vi "GUI - Template.vi"(5 "error in (no error)":errorcluster, 6 "ReInit All to Default?":bool, 7 "Application Name":string="GenUtil", 9 "State Queue":T1[](array[typedef])=["SC >>> Initialize"]) -> (19 "error out":errorcluster)   [LabVIEW 2020, in "Generic Utilities.lvclass"]
uses:
  Generic Utilities.lvclass
  utils/GenUtil State List.ctl
  <vilib>/Utility/sysdir.llb/System Directory Type.ctl
  <vilib>/Platform/browser.llb/Open URL in Default Browser (path).vi
  <vilib>/addons/_AddQ/G#Object/G#Object.lvclass
panel:
  in  "Task":enum32{"Monitor", "Settings"}(tab)
  in  "AppData Folder":bool
  out "State History":string[](array[string])
  out "State Index":i32
  out "Exec Time":dbl
  in  "TimeOut":i32=-1 caption="msec"
  in  "State 1":bool
  in  "Exit":bool
  # "Ó 2016"
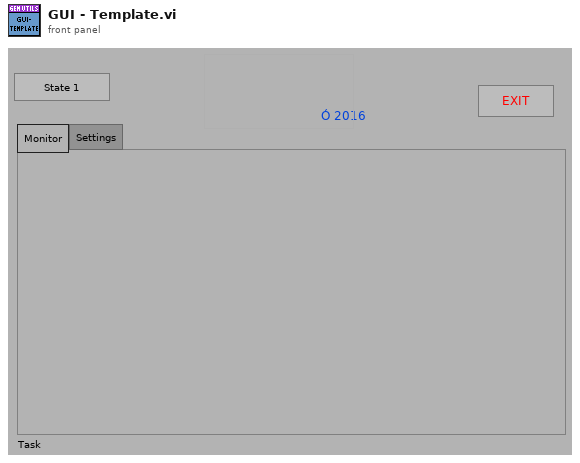
[diagram p1: front panel]
types:
  T1 = typedef "Generic Utilities.lvclass/GenUtil State List.ctl" = string
  T2 = enum32{"Invalid", "Standard", "Closed", "Hidden", "Minimized", "Maximized"}
  T3 = typedef "System Directory Type.ctl" = i32
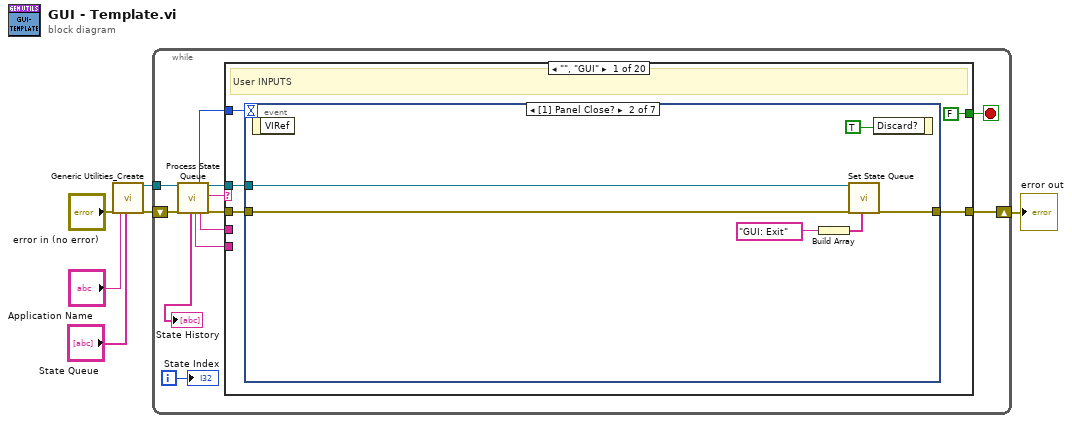
[diagram p0: block diagram]
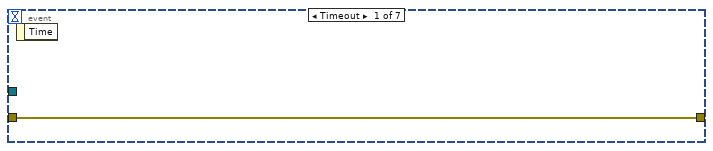
[diagram p2: hidden frame]
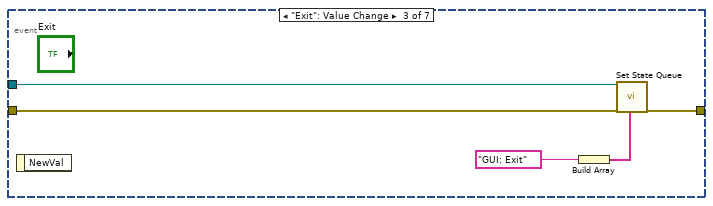
[diagram p3: hidden frame]
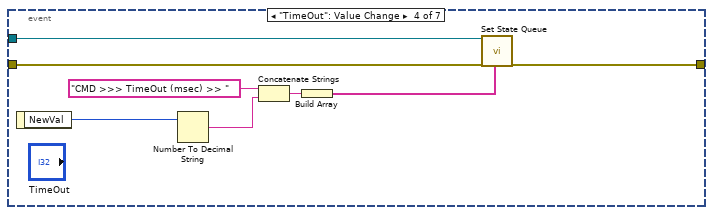
[diagram p4: hidden frame]
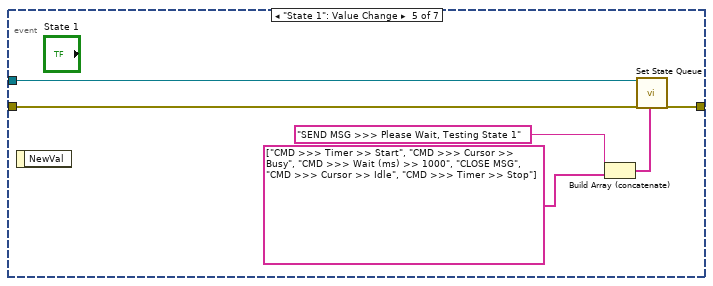
[diagram p5: hidden frame]
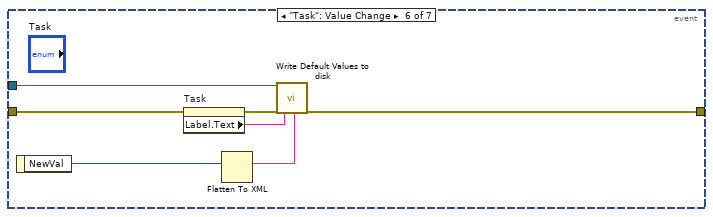
[diagram p6: hidden frame]
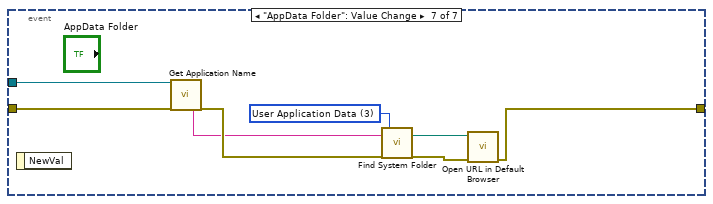
[diagram p7: hidden frame]
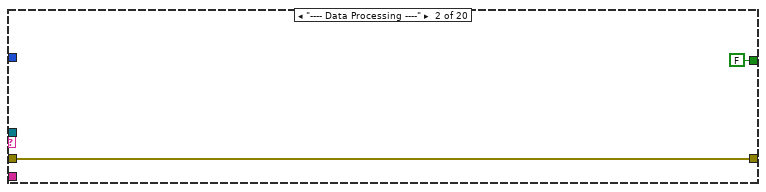
[diagram p8: hidden frame]
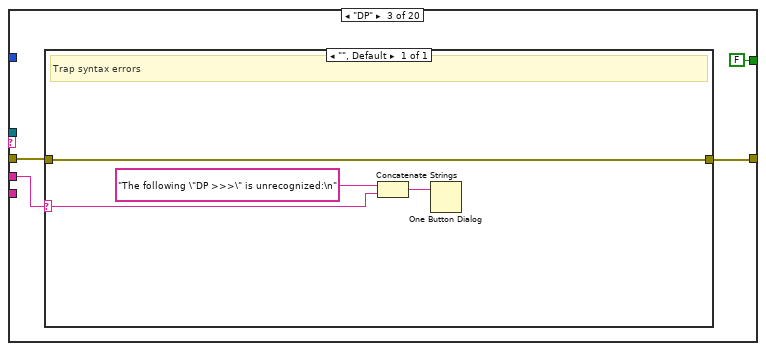
[diagram p9: hidden frame]
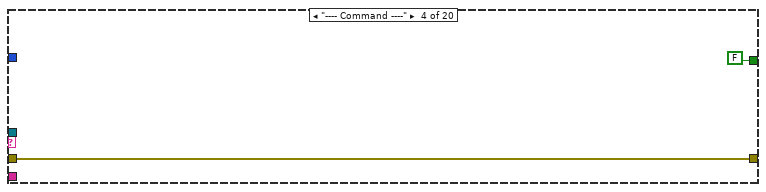
[diagram p10: hidden frame]
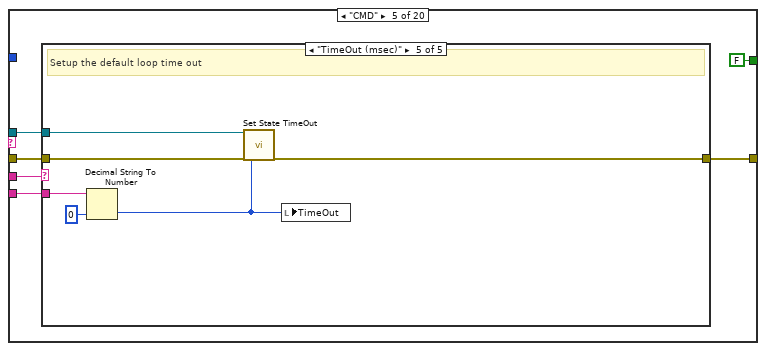
[diagram p11: hidden frame]
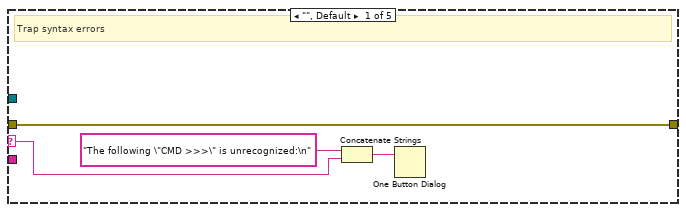
[diagram p12: hidden frame]
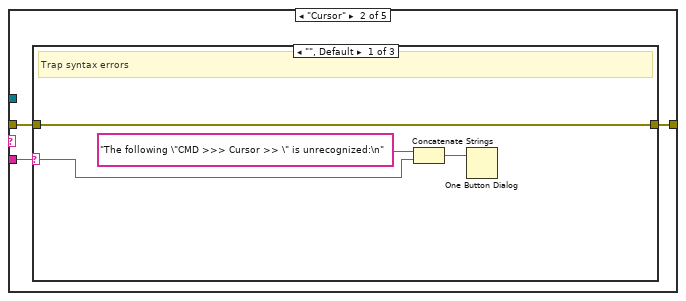
[diagram p13: hidden frame]
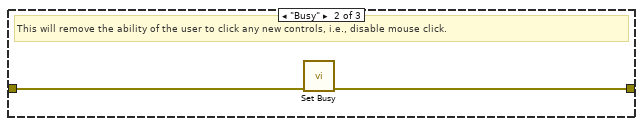
[diagram p14: hidden frame]
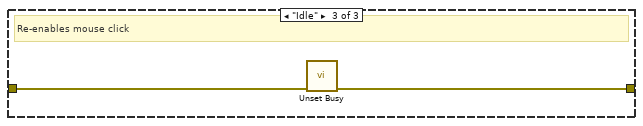
[diagram p15: hidden frame]
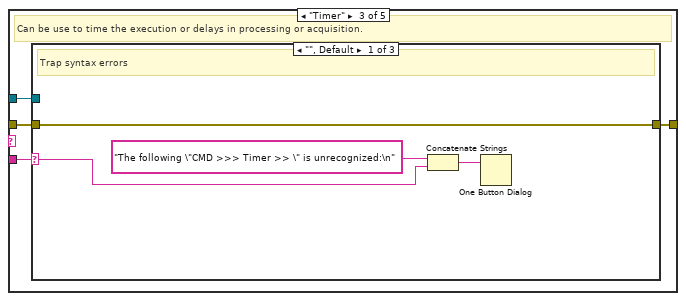
[diagram p16: hidden frame]
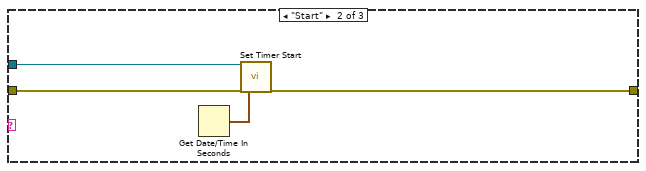
[diagram p17: hidden frame]
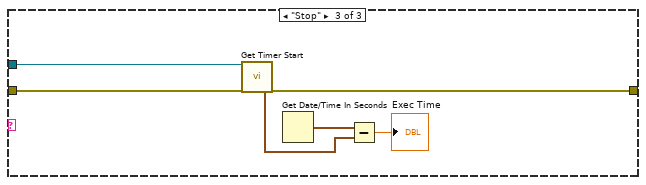
[diagram p18: hidden frame]
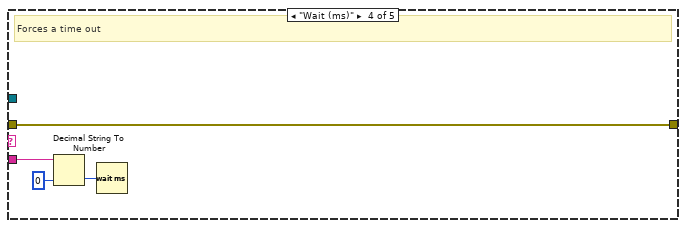
[diagram p19: hidden frame]
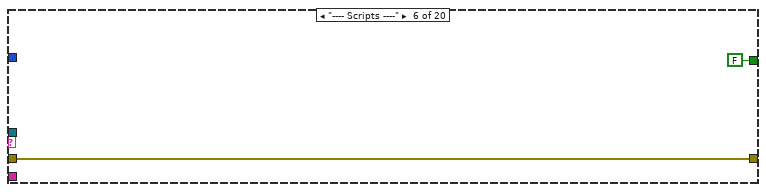
[diagram p20: hidden frame]
diagram:
  n1 = call "Generic Utilities_Create.vi"("error in (no error)"="error in (no error)", "Application Name"="Application Name", "State Queue"="State Queue") -> ("reference out"=w6:refnum<class "Generic Utilities.lvclass">, "error out"=w5:errorcluster)  [unwired: 15 in]
  n2 = while {
    shift-right: [w10] -> w1
    shift-left: w5 -> [w15]
    tunnel: w6 -> [w16]
    i -> [w17]
    stop <- w18 stop-if-true
    n3 = call "Process State Queue.vi"("reference in"=w16, "error in (no error)"=w15) -> ("State History"=→"State History":string[], "Additional Options"=w7:string, "Timeout"=w14:i32, "State Option"=w9:string, "reference out"=w13:refnum<class "Generic Utilities.lvclass">, "Current State"=w12:string, "error out"=w11:errorcluster)  [unwired: 10 in, 1 out]
    n4 = case shown="\"\", \"GUI\"" w12 {
      selector: w12 -> [_ _ _ _ _ _ _ _ _ _ _ _ _ _ _ _ w259 _ _ _]
      tunnel: w13 -> [w21 _ _ _ w77 _ w133 _ w144 w169 _ w199 w213 w248 w252 _ _ _ _ w269]
      tunnel: [FALSE FALSE FALSE FALSE FALSE FALSE FALSE FALSE FALSE FALSE FALSE FALSE TRUE FALSE FALSE FALSE FALSE FALSE FALSE TRUE] -> w18
      tunnel: w14 -> [w22 _ _ _ _ _ _ _ _ _ _ _ _ _ _ _ _ _ _ _]
      tunnel: w9 -> [_ _ w69 _ w81 _ w129 _ w145 w166 _ _ _ w245 _ _ _ _ _ _]
      tunnel: w11 -> [w20 w65 w68 w75 w79 w126 w132 w140 w142 w168 w189 w195 w210 w247 w253 w255 w257 w262 w265 w268]
      tunnel: [w19 w65 w67 w75 w80 w126 w131 w140 w143 w167 w189 w196 w209 w246 w251 w255 w257 errorcluster {"status"=FALSE, "code"=0, "source"=""} ("error out") w265 w267] -> w10
      tunnel: w7 -> [_ _ _ _ w78 _ _ _ _ _ _ _ _ _ _ _ _ _ _ _]
      frame "", "GUI" {
        # "User INPUTS"
        n5 = event shown="[1] Panel Close?" {
          selector: _ -> [_ _ _ _ _ _ _]
          dyn-events: _ -> [_ _ _ _ _ _ _]
          timeout: w22 -> [_ _ _ _ _ _ _]
          tunnel: w21 -> [_ w29 w35 w39 w48 w55 w63]
          tunnel: w20 -> [w24 w28 w33 w38 w47 w52 w62]
          tunnel: [w24 w27 w34 w37 w49 w50 w57] -> w19
          event Timeout {
            n6 = event-data() -> ()  [unwired: 1 in, 1 out]
          }
          event Panel Close? {
            n7 = event-data() -> ()  [unwired: 1 in, 1 out]
            n8 = Build Array(T1 "GUI: Exit" ("State List")) -> (w26:T1[])
            n9 = call "Set State Queue.vi"("reference in"=w29, "error in (no error)"=w28, "State Queue"=w26) -> ("error out"=w27:errorcluster)  [unwired: 15 in, 1 out]
            n10 = event-data("Discard?"=TRUE) -> ()  [unwired: 1 in, 1 out]
          }
          event "Exit": Value Change {
            n11 = event-data() -> ()  [unwired: 1 in, 1 out]
            n12 = Build Array(T1 "GUI: Exit" ("State List")) -> (w32:T1[])
            n13 = call "Set State Queue.vi"("reference in"=w35, "error in (no error)"=w33, "State Queue"=w32) -> ("error out"=w34:errorcluster)  [unwired: 15 in, 1 out]
          }
          event "TimeOut": Value Change {
            n14 = event-data() -> ("NewVal"=w36:i32)  [unwired: 1 in]
            n15 = Number To Decimal String(number=w36) -> (decimal integer string=w41:string)  [unwired: 1 in]
            n16 = Concatenate Strings("CMD >>> TimeOut (msec) >> " ("String"), w41) -> (w42:string)
            n17 = Build Array(w42) -> (w43:string[])
            n18 = call "Set State Queue.vi"("reference in"=w39, "error in (no error)"=w38, "State Queue"=w43) -> ("error out"=w37:errorcluster)  [unwired: 15 in, 1 out]
          }
          event "State 1": Value Change {
            n19 = event-data() -> ()  [unwired: 1 in, 1 out]
            n20 = Build Array (concatenate)("SEND MSG >>> Please Wait, Testing State 1" ("String"), T1[] ["CMD >>> Timer >> Start", "CMD >>> Cursor >> Busy", "CMD >>> Wait (ms) >> 1000", "CLOSE MSG", "CMD >>> Cursor >> Idle", "CMD >>> Timer >> Stop"] ("State Queue OUT")) -> (w44:T1[])
            n21 = call "Set State Queue.vi"("reference in"=w48, "error in (no error)"=w47, "State Queue"=w44) -> ("error out"=w49:errorcluster)  [unwired: 15 in, 1 out]
          }
          event "Task": Value Change {
            n22 = event-data() -> ("NewVal"=w56:enum32{"Monitor", "Settings"})  [unwired: 1 in]
            n23 = property on="Task" class="TabCtl (strict)"(error in=w52) -> (error out=w51:errorcluster, "Label.Text"=w54:string)  [unwired: 1 in, 1 out]
            n24 = Flatten To XML(6:w56) -> (2:w53:string)
            n25 = call-dynamic "Write Default Values to disk.vi"("reference in"=w55, "error in (no error)"=w51, "Control Label"=w54, "Value (XML String)"=w53) -> ("error out"=w50:errorcluster)  [unwired: 14 in, 1 out]
          }
          event "AppData Folder": Value Change {
            w64 = T3 3 items=["User Home"=0, "User Desktop"=1, "User Documents"=2, "User Application Data"=3, "User Preferences"=4, "User Temporary"=5, "Public Documents"=6, "Public Application Data"=7, "Public Preferences"=8, "Public Cache"=13, "System Core Libraries"=9, "System Installed Libraries"=10, "Application Files"=11, "Boot Volume Root"=12] ("system directory type")
            n26 = event-data() -> ()  [unwired: 1 in, 1 out]
            n27 = call "Get Application Name.vi"("reference in"=w63, "error in (no error)"=w62) -> ("Application Name"=w60:string, "error out"=w61:errorcluster)  [unwired: 15 in, 1 out]
            n28 = call "Find System Folder.vi"("Application Name"=w60, "error in (no error)"=w61, "system directory type"=w64) -> ("System Folder"=w59:path, "error out"=w58:errorcluster)  [unwired: 15 in]
            n29 = call-poly <vilib>:"Open URL in Default Browser.vi"("error in (no error)"=w58, "path"=w59) -> ("error out"=w57:errorcluster)  [unwired: 4 in, 1 out]
          }
        }
      }
      frame "---- Data Processing ----" {
      }
      frame "DP" {
        n30 = case shown="\"\", Default" w69 {
          selector: w69 -> [w72]
          tunnel: [w71] -> w67
          tunnel: w68 -> [w71]
          frame "", Default {
            # "Trap syntax errors"
            n31 = Concatenate Strings("The following \"DP >>>\" is unrecognized:\n", w72) -> (w73:string)
            n32 = One Button Dialog(message=w73) -> ()  [unwired: 1 in, 1 out]
          }
        }
      }
      frame "---- Command ----" {
      }
      frame "CMD" {
        n33 = case shown="\"TimeOut (msec)\"" w81 {
          selector: w81 -> [w84 _ _ _ _]
          tunnel: [w83 w88 w100 w119 w121] -> w80
          tunnel: w79 -> [w83 w87 w99 w119 w122]
          tunnel: w78 -> [_ w89 w101 w116 w124]
          tunnel: w77 -> [_ _ w98 _ w123]
          frame "", Default {
            # "Trap syntax errors"
            n34 = Concatenate Strings("The following \"CMD >>>\" is unrecognized:\n", w84) -> (w85:string)
            n35 = One Button Dialog(message=w85) -> ()  [unwired: 1 in, 1 out]
          }
          frame "Cursor" {
            n36 = case shown="\"\", Default" w89 {
              selector: w89 -> [w91 _ _]
              tunnel: [w90 w94 w96] -> w88
              tunnel: w87 -> [w90 w95 w97]
              frame "", Default {
                # "Trap syntax errors"
                n37 = Concatenate Strings("The following \"CMD >>> Cursor >> \" is unrecognized:\n", w91) -> (w92:string)
                n38 = One Button Dialog(message=w92) -> ()  [unwired: 1 in, 1 out]
              }
              frame "Busy" {
                # "This will remove the ability of the user to click any new controls, i.e., disable mouse click."
                n39 = call <vilib>:"Set Busy.vi"("error in (no error)"=w95) -> ("error out"=w94:errorcluster)  [unwired: 9 in, 1 out]
              }
              frame "Idle" {
                # "Re-enables mouse click"
                n40 = call <vilib>:"Unset Busy.vi"("error in (no error)"=w97) -> ("error out"=w96:errorcluster)  [unwired: 10 in]
              }
            }
          }
          frame "Timer" {
            # "Can be use to time the execution or delays in processing or acquisition."
            n41 = case shown="\"\", Default" w101 {
              selector: w101 -> [w103 _ _]
              tunnel: [w102 w107 w112] -> w100
              tunnel: w99 -> [w102 w108 w113]
              tunnel: w98 -> [_ w109 w114]
              frame "", Default {
                # "Trap syntax errors"
                n42 = Concatenate Strings("The following \"CMD >>> Timer >> \" is unrecognized:\n", w103) -> (w104:string)
                n43 = One Button Dialog(message=w104) -> ()  [unwired: 1 in, 1 out]
              }
              frame "Start" {
                n44 = Get Date/Time In Seconds() -> (seconds since 1Jan1904=w106:timestamp)
                n45 = call "Set Timer Start.vi"("reference in"=w109, "error in (no error)"=w108, "Timer Start"=w106) -> ("error out"=w107:errorcluster)  [unwired: 15 in, 1 out]
              }
              frame "Stop" {
                n46 = call "Get Timer Start.vi"("reference in"=w114, "error in (no error)"=w113) -> ("Timer Start"=w111:timestamp, "error out"=w112:errorcluster)  [unwired: 15 in, 1 out]
                n47 = Get Date/Time In Seconds() -> (seconds since 1Jan1904=w115:timestamp)
                n48 = Subtract(x=w115, y=w111) -> (x-y=→"Exec Time":dbl)
              }
            }
          }
          frame "Wait (ms)" {
            # "Forces a time out"
            n49 = Decimal String To Number(string=w116, default (0L)=u32 0 ("default (0 I32)")) -> (number=w117:u32)  [unwired: 1 in, 1 out]
            n50 = Wait (ms)(milliseconds to wait=w117) -> ()  [unwired: 1 out]
          }
          frame "TimeOut (msec)" {
            # "Setup the default loop time out"
            n51 = Decimal String To Number(string=w124, default (0L)=0 ("default (0 I32)")) -> (number=w120:i32)  [unwired: 1 in, 1 out]
            n52 = call "Set State TimeOut.vi"("reference in"=w123, "error in (no error)"=w122, "TimeOut (msec)"=w120) -> ("error out"=w121:errorcluster)  [unwired: 15 in, 1 out]
            n53 = local write "TimeOut"(w120) -> ()
          }
        }
      }
      frame "---- Scripts ----" {
      }
      frame "SC" {
        n54 = case shown="\"Initialize\"" w129 {
          selector: w129 -> [w136 _]
          tunnel: [string[] [] ("State Queue OUT") string[] ["GUI: Initialize Ref", "CTRL >>> Task Tab", "FP >>> Open"] ("State Queue OUT")] -> w130
          frame "False", Default {
            n55 = Concatenate Strings("The following \"Script\" is unrecognized:\n", w136) -> (w137:string)
            n56 = One Button Dialog(message=w137) -> ()  [unwired: 1 in, 1 out]
          }
          frame "Initialize" {
          }
        }
        n57 = call "Set State Queue.vi"("reference in"=w133, "error in (no error)"=w132, "State Queue Options"=enum16{"Replace", "Append", "Prepend"}."Prepend", "State Queue"=w130) -> ("error out"=w131:errorcluster)  [unwired: 14 in, 1 out]
      }
      frame "---- Front Panel Mgmt ----" {
      }
      frame "CTRL" {
        n58 = case shown="\"Task Tab\"" w145 {
          selector: w145 -> [w149 _]
          tunnel: w144 -> [_ w157]
          tunnel: [w147 w153] -> w143
          tunnel: w142 -> [w147 w155]
          frame "unknown", Default {
            n59 = Concatenate Strings("The following control name is unrecognized:\n", w149) -> (w148:string)
            n60 = One Button Dialog(message=w148) -> ()  [unwired: 1 in, 1 out]
          }
          frame "Task Tab" {
            n61 = property on="Task" class="TabCtl (strict)"(error in=w155) -> (error out=w156:errorcluster, "Label.Text"=w154:string, "Value"=w158:enum32{"Monitor", "Settings"})  [unwired: 1 in, 1 out]
            n62 = call-dynamic "Read Default Values from Disk.vi"("reference in"=w157, "error in (no error)"=w156, "Control Label"=w154) -> ("Value (XML String)"=w152:string, "error out"=w151:errorcluster)  [unwired: 14 in, 1 out]
            n63 = case shown="\"anything\", Default" w152 {
              selector: w152 -> [w164 _]
              tunnel: [w160 w165] -> w159
              tunnel: w158 -> [w162 w165]
              frame "anything", Default {
                # "Decode XML"
                n64 = Unflatten From XML(xml string=w164, type=w162) -> (value=w161:enum32{"Monitor", "Settings"}, error out=w163:errorcluster)  [unwired: 1 in]
                n65 = Select(t=w162, s=w163, f=w161) -> (s? t:f=w160:enum32{"Monitor", "Settings"})
              }
              frame "" {
                # "NO File / Error"
              }
            }
            n66 = property on="Task" class="TabCtl (strict)"(error in=w151, "Value"=w159) -> (error out=w153:errorcluster)  [unwired: 1 in, 1 out]
          }
        }
      }
      frame "FP" {
        n67 = case shown="\"Open\"" w166 {
          selector: w166 -> [w171 _]
          tunnel: w169 -> [_ w179]
          tunnel: w168 -> [w172 w178]
          tunnel: [w172 w175] -> w167
          frame "unknown", Default {
            n68 = Concatenate Strings("The following FP Command name is unrecognized:\n", w171) -> (w173:string)
            n69 = One Button Dialog(message=w173) -> ()  [unwired: 1 in, 1 out]
          }
          frame "Open" {
            n70 = call-dynamic "Get VI Ref.vi"("reference in"=w179, "error in (no error)"=w178) -> ("GUI VI Ref"=w176:refnum<vi>, "error out"=w177:errorcluster)  [unwired: 14 in, 2 out]
            n71 = property class="VI"(reference=w176, error in=w177) -> (reference out=w181:refnum<vi>, error out=w182:errorcluster, "Front Panel.Open"=w180:bool)
            n72 = case shown="False" w180 {
              tunnel: [w185 w188] -> w175
              tunnel: w182 -> [w184 w188]
              tunnel: w181 -> [w183 _]
              frame False {
                n73 = invoke class="VI" method="FP.Open"(reference=w183, error in=w184, "Activate"=TRUE, "State"=T2."Standard") -> (error out=w185:errorcluster)  [unwired: 1 in, 4 out]
              }
              frame True {
              }
            }
          }
        }
      }
      frame "---- GUI Functions ----" {
      }
      frame "GUI: Initialize Ref" {
        n74 = control-ref of="GUI Reference"() -> (w194:refnum<vi>)
        n75 = call "Set VI Ref.vi"("reference in"=w199, "error in (no error)"=w195, "ReInit All to Default?"="ReInit All to Default?", "GUI VI Ref"=w194) -> ("reference out"=w198:refnum<class "Generic Utilities.lvclass">, "error out"=w193:errorcluster)  [unwired: 14 in]
        n76 = call "Set Close Panel (Yes or No).vi"("reference in"=w198, "error in (no error)"=w193) -> ("reference out"=w197:refnum<class "Generic Utilities.lvclass">, "error out"=w192:errorcluster)  [unwired: 16 in]
        n77 = call "Set Message Window Ref.vi"("reference in"=w197, "error in (no error)"=w192) -> ("error out"=w196:errorcluster)  [unwired: 16 in, 1 out]
      }
      frame "GUI: Exit" {
        n78 = call-dynamic "Get Message Window Ref.vi"("reference in"=w213, "error in (no error)"=w210) -> ("reference out"=w212:refnum<class "Generic Utilities.lvclass">, "Msg Win Ref"=w208:refnum<vi>, "error out"=w211:errorcluster)  [unwired: 15 in]
        n79 = call-dynamic "Get VI Ref.vi"("reference in"=w212, "error in (no error)"=w211) -> ("reference out"=w216:refnum<class "Generic Utilities.lvclass">, "GUI VI Ref"=w214:refnum<vi>, "error out"=w215:errorcluster)  [unwired: 14 in, 1 out]
        n80 = local write "Exit"(FALSE ("Exit")) -> ()
        n81 = call-dynamic "Get Close Panel (Yes or No).vi"("reference in"=w216, "error in (no error)"=w215) -> ("Close Panel?"=w217:bool, "reference out"=w206:refnum<class "Generic Utilities.lvclass">, "error out"=w207:errorcluster)  [unwired: 15 in]
        n82 = call-dynamic "Get OBJ NOT RefNum.vi"("reference in"=w206, "error in (no error)"=w207) -> ("OBJ not a refnum?"=w205:bool, "reference out"=w204:refnum<class "Generic Utilities.lvclass">, "error out"=w203:errorcluster)  [unwired: 15 in]
        n83 = case shown="True" w205 {
          tunnel: [w222 w225] -> w202
          tunnel: w204 -> [_ w224]
          tunnel: w203 -> [w222 w223]
          frame False {
            # "The OBJ already exist, indicating this is a dialog box or sub-vi so do NOT destroy the original OBJ."
          }
          frame True {
            # "New OBJ was created, so it needs to be deleted."
            n84 = call-dynamic "Destroy.vi"("reference in"=w224, "error in (no error)"=w223) -> ("error out"=w226:errorcluster)  [unwired: 16 in, 1 out]
            n85 = disable-structure shown="Disabled" {
              disable-tunnel: w226 -> [w228 w229]
              disable-tunnel: [w227 w229] -> w225
              frame Disabled {
                # "Enable when NEEDED"
                n86 = call <vilib>:"GarbageCollector.vi"("error in (no error)"=w228) -> ("error out"=w227:errorcluster)  [unwired: 16 in, 2 out]
              }
              frame Enabled {
              }
            }
          }
        }
        n87 = Close Reference(reference=w208, error in (no error)=w202) -> (error out=w220:errorcluster)
        n88 = case shown="True" w217 {
          tunnel: w220 -> [w231 w235]
          tunnel: [w231 w234] -> w218
          tunnel: [w230 w233] -> w219
          tunnel: w214 -> [w230 w232]
          frame False {
          }
          frame True {
            n89 = property class="VI"(reference=w232, error in=w235) -> (reference out=w237:refnum<vi>, error out=w236:errorcluster, "Front Panel.Open"=w238:bool)
            n90 = case shown="True" w238 {
              tunnel: [w240 w244] -> w234
              tunnel: w236 -> [w240 w243]
              tunnel: w237 -> [w239 w242]
              tunnel: [w239 w241] -> w233
              frame False {
              }
              frame True {
                n91 = invoke class="VI" method="FP.Close"(reference=w242, error in=w243) -> (reference out=w241:refnum<vi>, error out=w244:errorcluster)  [unwired: 1 in, 1 out]
              }
            }
          }
        }
        n92 = Close Reference(reference=w219, error in (no error)=w218) -> (error out=w209:errorcluster)
      }
      frame "SEND MSG" {
        n93 = call-dynamic "Send Message.vi"("reference in"=w248, "error in (no error)"=w247, "Message (\"\" closes the window)"=w245) -> ("error out"=w246:errorcluster)  [unwired: 15 in, 1 out]
      }
      frame "CLOSE MSG" {
        n94 = call-dynamic "Send Message.vi"("reference in"=w252, "error in (no error)"=w253, "Message (\"\" closes the window)"="Close" ("Message")) -> ("error out"=w251:errorcluster)  [unwired: 15 in, 1 out]
      }
      frame "---- Miscelleneous ----" {
      }
      frame "unknown", Default {
        n95 = Concatenate Strings("The following state is unrecognized?\n", w259) -> (w258:string)
        n96 = One Button Dialog(message=w258) -> ()  [unwired: 1 in, 1 out]
      }
      frame "Error" {
        n97 = call <vilib>:"General Error Handler.vi"("error in (no error)"=w262) -> ()  [unwired: 10 in, 5 out]
      }
      frame "Next" {
        # "This is an empty case used so the queue does NOT stop if there is an empty string between two valid states!"
      }
      frame "Quit" {
        # "WARNING!, If the state machine crash, then it will also \"Quit\"??"
        # "This is the case used to simply exit when this GUI is used as a SubVI!"
        n98 = call-dynamic "Destroy.vi"("reference in"=w269, "error in (no error)"=w268) -> ("error out"=w267:errorcluster)  [unwired: 16 in, 1 out]
      }
    }
    "State Index" <- w17
  }
  "error out" <- w1
